vi "Z6_Beamline.ProcEvents.vi"(0 "i ref in":refnum<vi>, 5 "error in (no error)":errorcluster) -> (14 "i ref out":refnum<vi>, 19 "error out":errorcluster)   [LabVIEW 2014, in "Z6_Beamline.lvlib"]
doc: "This method is used to define the events the object will listen to. Add your own events here."
uses:
  Z6_Beamline.lvlib
  PH_Beamline_Chief/PH_Beamline_Chief.Section.ctl
  CSCore/BaseProcess/BaseProcess.lvlib
  PH_Common/PH_Common.lvlib
  PH_Beamline_Chief/PH_Beamline_Chief.lvlib
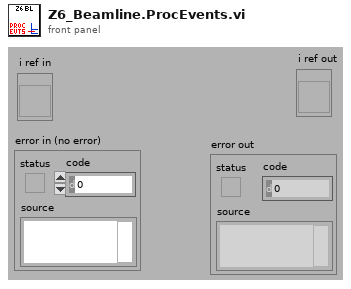
[diagram p1: front panel]
types:
  T1 = typedef "PH_Beamline_Chief.lvlib/PH_Beamline_Chief.Section.ctl" = enum16{"None", "YLF", "fs", "fs-YLF", "ns", "PA-Input", "PA-Undelay", "PA-Delay", "PA-before-Bypass", "PA", "PA-Bypass", "PA-Exit", "PA-LL", "LL", "PA-MA", "MA-Exit", "MA-Z6", "Z6", "MA-LB", "LB-TB2", "LB-TB3"}
  T2 = typedef "PH_Common.lvlib/PH_DIM.Event Declarer.ctl" = cluster{"Service Name":string, "Selector":string}
  T3 = typedef "BaseProcess.lvlib/BaseProcess.event definition.ctl" = cluster{"CAEEvtDef":T4, "Data Descriptor":T5}
  T4 = typedef "CAEObj.lvlib/CAEObj.event definition.ctl" = cluster{"URL":string, "enable":bool, "ignoreResID":bool}
  T5 = typedef "BaseProcess.lvlib/BaseProcess.descriptor string definition.ctl" = string
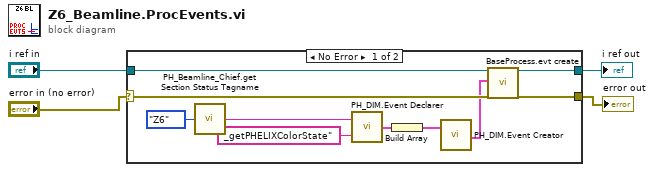
[diagram p0: block diagram]
diagram:
  n1 = case shown="No Error" "error in (no error)" {
    selector: "error in (no error)" -> [w10 w15]
    tunnel: [w14 w15] -> w4
    tunnel: [w13 w16] -> w3
    tunnel: "i ref in" -> [w9 w16]
    frame No Error {
      n2 = call "PH_Beamline_Chief.get Section Status Tagname.vi"("Beamline Section"=PH_Beamline_Chief.Section."Z6") -> ("Section Status Tagname"=w8:string)
      n3 = call "PH_DIM.Event Declarer.vi"("Selector"="_getPHELIXColorState", "Service Name"=w8) -> ("declared DIM Event"=w7:T2)
      n4 = Build Array(w7) -> (w5:T2[])
      n5 = call "PH_DIM.Event Creator.vi"("Trendmessage Services"=w5) -> ("DIM Service Events"=w6:T3[])  [unwired: 18 in]
      n6 = call "BaseProcess.evt create.vi"("i ref in"=w9, "newEvents"=w6, "error in (no error)"=w10) -> ("i ref out"=w13:refnum<vi>, "error out"=w14:errorcluster)  [unwired: 13 in, 2 out]
    }
    frame Error {
    }
  }
  "i ref out" <- w3
  "error out" <- w4
